vi "sort standard.vi"(6 "which measurements":string[](array[string])=["average cycle ratio", "std seq counts", "std seq q", "std seq ratio", "std seq norm", "std internal error", "std internal error(%)", "std external error", "std external error(%)", "std error", "ext vs int"], 8 "error in":errorcluster, 10 "cycle results cluster in":T1) -> (0 "error out":errorcluster)   [LabVIEW 2016]
uses:
  controls/cycle results control.ctl
panel:
  out "error out 2":errorcluster
  out "Numeric":i32
  out "Array":dbl[][](array[numeric])
  out "cycle results dbl":dbl[][](array[numeric])
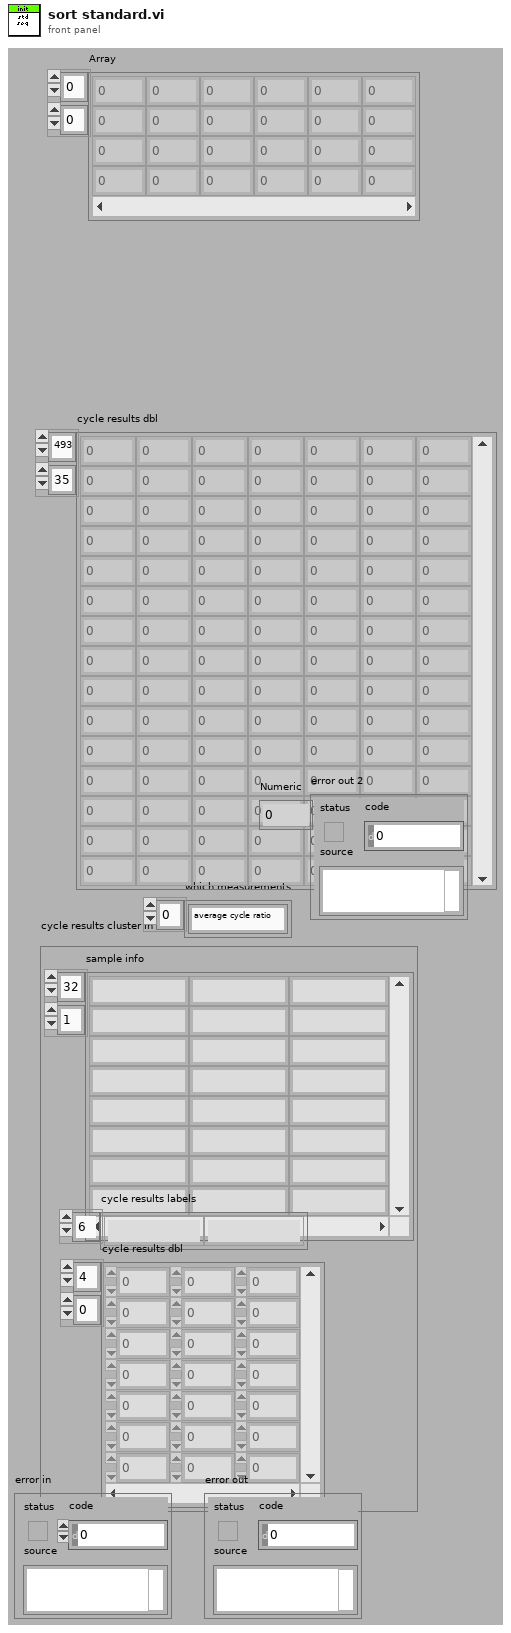
[diagram p1: front panel]
types:
  T1 = typedef "cycle results control.ctl" = cluster{"sample info":string[][], "cycle results labels":string[], "cycle results dbl":dbl[][]}
  T2 = typedef "data control cluster.ctl" = cluster{"Final result header":string[], "sequence result header":string[], "cycle result header ":string[], "Final Result":string[][], "sequence  Result":dbl[][], "Cycle data by seq":dbl[][][], "Cycle data by position":dbl[][][], "Final seq  Result":dbl[][], "only specific type":dbl[][]}
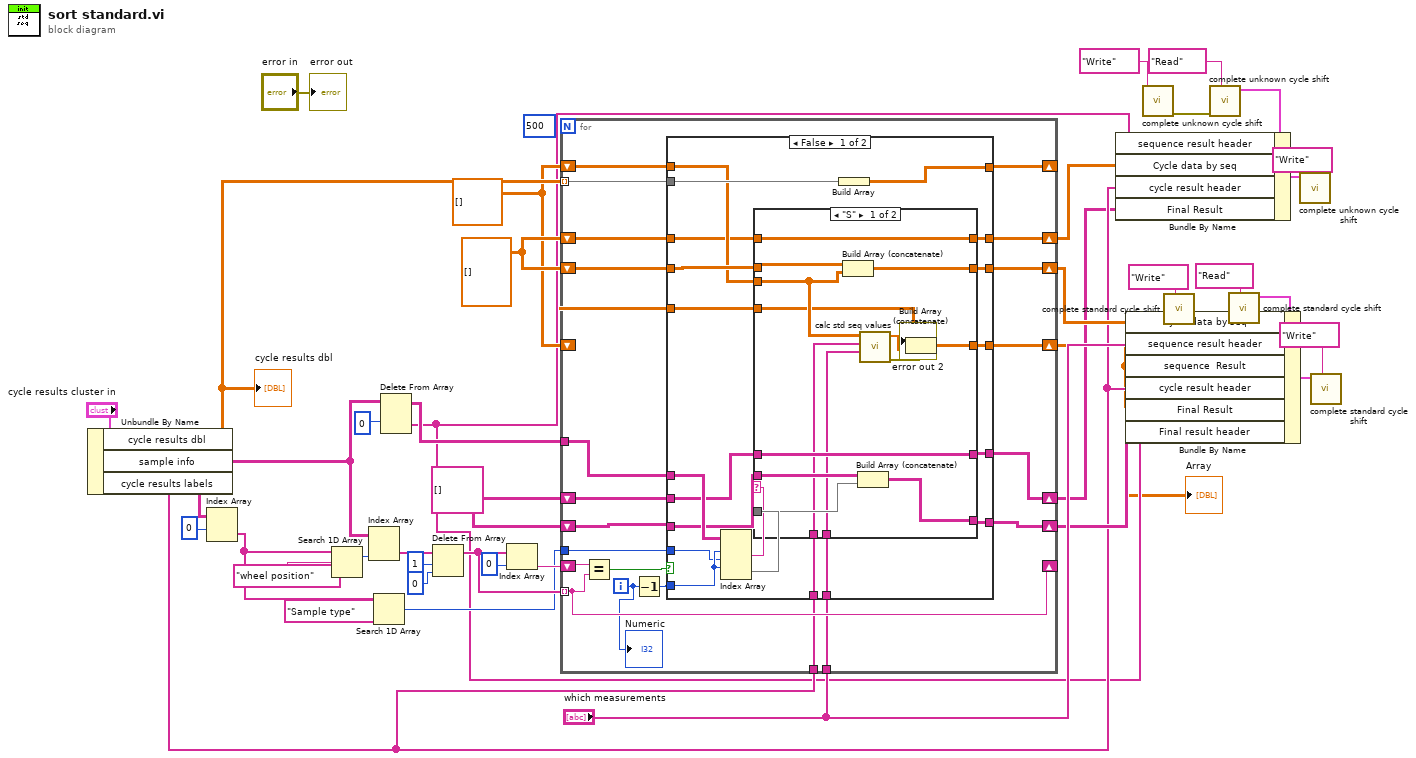
[diagram p0: block diagram]
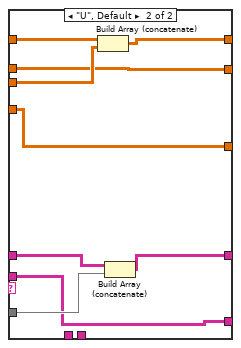
[diagram p2: hidden frame]
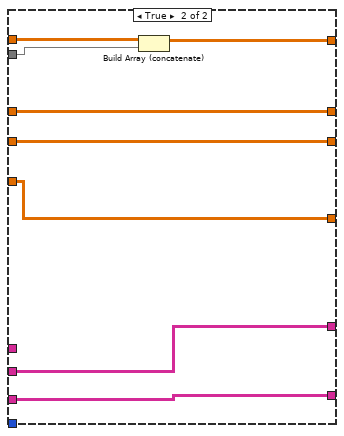
[diagram p3: hidden frame]
diagram:
  (unwired) 500
  w25 = dbl[][][] []
  w26 = string[][] []
  w21 = dbl[][] []
  n1 = Unbundle By Name("cycle results cluster in") -> ("cycle results dbl"=w24:dbl[][], "sample info"=w23:string[][], "cycle results labels"=w11:string[])
  "cycle results dbl" <- w24
  n2 = Index Array(array=w23, index (row)=0) -> (element=w29:string[])  [unwired: 1 in]
  n3 = Search 1D Array(1D array=w29, element="wheel position") -> (index of element=w30:i32)  [unwired: 1 in]
  n4 = Index Array(array=w23, index (col)=w30) -> (element=w36:string[])  [unwired: 1 in]
  n5 = Search 1D Array(1D array=w29, element="Sample type") -> (index of element=w27:i32)  [unwired: 1 in]
  n6 = Delete From Array(array=w23, index (row)=0) -> (deleted portion=w9:string[], array with subset deleted=w31:string[][])  [unwired: 2 in]
  n7 = Delete From Array(array=w36, length=1, index=0) -> (array with subset deleted=w35:string[])  [unwired: 1 out]
  n8 = Index Array(array=w35, index=0) -> (element=w33:string)
  n9 = for {
    tunnel: w35 -> [w47] mode=indexing
    tunnel: w24 -> [w62] mode=indexing
    shift-right: [w61] -> _
    shift-left: w21 -> [w60]
    shift-right: [w59] -> w15
    shift-left: w25 -> [w58]
    shift-right: [w56] -> w16
    shift-left: w26 -> [w55]
    tunnel: w31 -> [w54]
    shift-right: [w47] -> _
    shift-left: w33 -> [w48]
    tunnel: w27 -> [w53]
    shift-right: [w52] -> w8
    shift-left: w26 -> [w51]
    shift-right: [w50] -> w10
    shift-left: w25 -> [w49]
    shift-right: [w46] -> w4
    shift-left: w21 -> [w45]
    tunnel: "which measurements" -> [w44]
    tunnel: w11 -> [w43]
    i -> [w42]
    n10 = Equal?(x=w48, y=w47) -> (x = y?=w63:bool)
    n11 = Decrement(x=w42) -> (x-1=w57:i32)
    n12 = case shown="False" w63 {
      tunnel: w54 -> [w81 _]
      tunnel: w62 -> [w83 w114]
      tunnel: [w82 w113] -> w61
      tunnel: w60 -> [w78 w112]
      tunnel: [w77 w111] -> w59
      tunnel: w58 -> [w79 w111]
      tunnel: w57 -> [w80 _]
      tunnel: [w75 w110] -> w56
      tunnel: w55 -> [w76 w110]
      tunnel: w53 -> [w70 _]
      tunnel: [w74 w108] -> w52
      tunnel: w51 -> [w73 w108]
      tunnel: [w72 w109] -> w50
      tunnel: w49 -> [w71 w109]
      tunnel: [w67 w107] -> w46
      tunnel: w45 -> [w66 w107]
      tunnel: w44 -> [w65 _]
      tunnel: w43 -> [w64 _]
      frame False {
        n13 = Index Array(array=w81, index (row) #1=w80, index (col) #1=w70, index (row) #2=w80) -> (element #1=w68:string, element #2=w69:string[])  [unwired: 1 in]
        n14 = case shown="\"S\"" w68 {
          tunnel: w79 -> [w92 w99]
          tunnel: w78 -> [w90 w106]
          tunnel: [w97 w99] -> w77
          tunnel: w76 -> [w95 w102]
          tunnel: [w96 w102] -> w75
          tunnel: w69 -> [w91 w105]
          tunnel: [w94 w104] -> w74
          tunnel: w73 -> [w94 w103]
          tunnel: [w93 w101] -> w72
          tunnel: w71 -> [w93 w100]
          tunnel: [w89 w98] -> w67
          tunnel: w66 -> [w87 w98]
          tunnel: w65 -> [w86 _]
          tunnel: w64 -> [w85 _]
          frame "S" {
            n15 = Build Array (concatenate)(w92, w90) -> (w97:dbl[][][])
            n16 = Build Array (concatenate)(w95, w91) -> (w96:string[][])
            n17 = call "calc std seq values.vi"("which measurements"=w86, "cycle results labels"=w85, "std cycle results dbl"=w90) -> ("error out"=→"error out 2":errorcluster, "std seq results"=w88:dbl[])  [unwired: 7 in]
            n18 = Build Array (concatenate)(w87, w88) -> (w89:dbl[][])
          }
          frame "U", Default {
            n19 = Build Array (concatenate)(w100, w106) -> (w101:dbl[][][])
            n20 = Build Array (concatenate)(w103, w105) -> (w104:string[][])
          }
        }
        n21 = Build Array(w83) -> (w82:dbl[][])
      }
      frame True {
        n22 = Build Array (concatenate)(w112, w114) -> (w113:dbl[][])
      }
    }
    "Numeric" <- w42
  }
  "Array" <- w4
  n23 = call "complete unknown cycle shift.vi"("read write shift"="Write") -> ("error out"=w1:errorcluster)  [unwired: 9 in, 1 out]
  n24 = call "complete standard cycle shift.vi"("read write shift"="Write") -> ("error out"=w2:errorcluster)  [unwired: 9 in, 1 out]
  n25 = call "complete unknown cycle shift.vi"("read write shift"="Read", "error in"=w1) -> ("DATA CLUSTER out"=w12:T2)  [unwired: 8 in, 1 out]
  n26 = Bundle By Name(cluster=w12, "sequence result header"=w9, "Cycle data by seq"=w10, "cycle result header"=w11, "Final Result"=w8) -> (w6:T2)
  n27 = call "complete standard cycle shift.vi"("read write shift"="Read", "error in"=w2) -> ("DATA CLUSTER out"=w18:T2)  [unwired: 8 in, 1 out]
  n28 = Bundle By Name(cluster=w18, "Cycle data by seq"=w15, "sequence result header"="which measurements", "sequence  Result"=w4, "cycle result header"=w11, "Final Result"=w16, "Final result header"=w9) -> (w7:T2)
  n29 = call "complete unknown cycle shift.vi"("read write shift"="Write", "DATA CLUSTER in"=w6) -> ()  [unwired: 8 in, 2 out]
  n30 = call "complete standard cycle shift.vi"("read write shift"="Write", "DATA CLUSTER in"=w7) -> ()  [unwired: 8 in, 2 out]
  "error out" <- "error in"
